vi "Fit Transform.vi"(7 "Type X":T1(ring), 8 "error in (no error)":errorcluster caption="entrée d'erreur (pas d'erreur)", 10 "y":string[][](array[string]), 11 "LabelBinarizer.lvclass":refnum<class "LabelBinarizer.lvclass">) -> (0 "error out":errorcluster caption="sortie d'erreur", 2 "Data":T2, 3 "LabelBinarizer.lvclass":refnum<class "LabelBinarizer.lvclass">)   [LabVIEW 2020, in "LabelBinarizer.lvclass"]
doc: "Fit label binarizer and transform multi-class labels to binary labels.\n\nThe output of transform is sometimes referred to as the 1-of-K coding scheme.\n\nReturns : \n\n- Y : array or CSR matrix of shape [n_samples, n_classes]\nShape will be [n_samples, 1] for binary problems."
uses:
  LabelBinarizer.lvclass
  LabelBinarizer.lvclass/LabelBinarizer.ctl
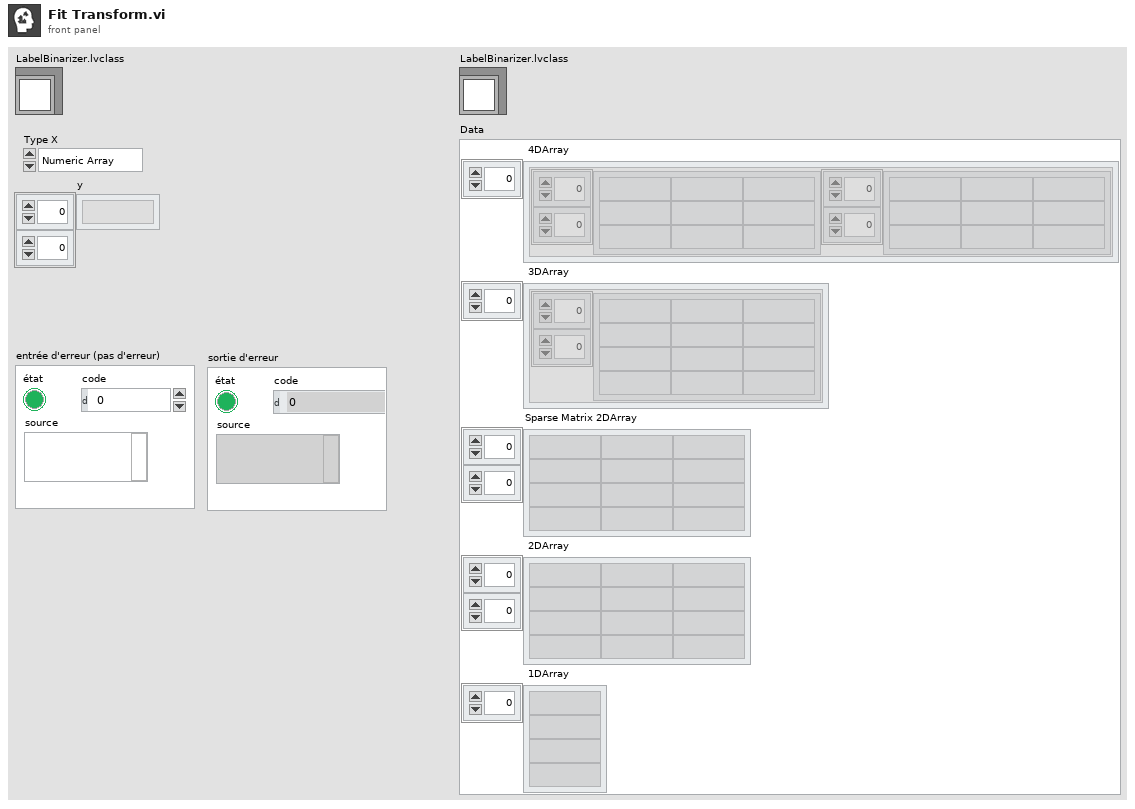
[diagram p1: front panel]
types:
  T1 = enum16{"Numeric Array", "String Array", "Sparse"}
  T2 = cluster{" 4DArray":cluster{"1":string[][], "2":string[][]}[], " 3DArray":cluster{"Tableau":string[][]}[], "Sparse Matrix 2DArray":string[][], " 2DArray":string[][], " 1DArray":string[]}
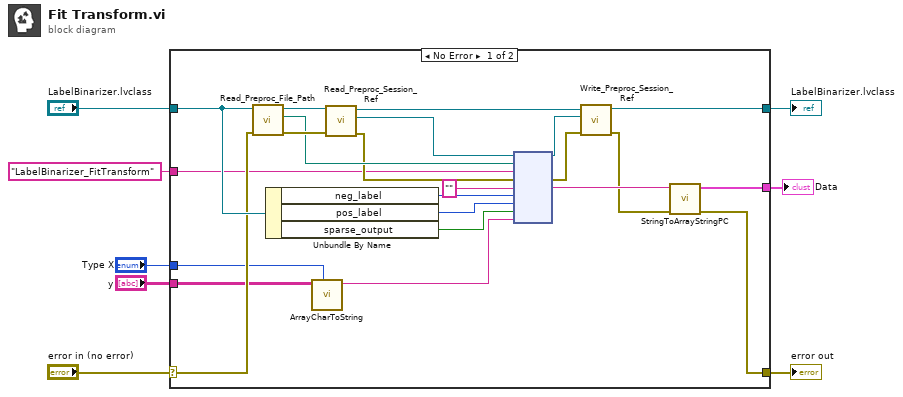
[diagram p0: block diagram]
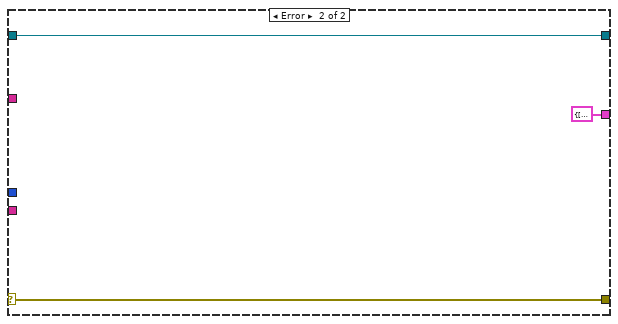
[diagram p2: hidden frame]
diagram:
  n1 = case shown="No Error" "error in (no error)" {
    selector: "error in (no error)" -> [w18 w34]
    tunnel: [w9 w34] -> w7
    tunnel: [w11 w33] -> w5
    tunnel: "LabelBinarizer.lvclass" -> [w19 w33]
    tunnel: "LabelBinarizer_FitTransform" ("Fonction") -> [w17 _]
    tunnel: [w10 T2 {" 4DArray"=[], " 3DArray"=[], "Sparse Matrix 2DArray"=[], " 2DArray"=[], " 1DArray"=[]} ("Data")] -> w3
    tunnel: "y" -> [w16 _]
    tunnel: "Type X" -> [w15 _]
    frame No Error {
      n2 = call-dynamic "Read_Preproc_File_Path.vi"("error in (no error)"=w18, "Python in"=w19) -> ("error out"=w30:errorcluster, "File_Path"=w27:path, "Python out"=w31:refnum<class "LabelBinarizer.lvclass">)  [unwired: 7 in]
      n3 = Unbundle By Name(w19) -> ("neg_label"=w22:i32, "pos_label"=w21:i32, "sparse_output"=w20:bool)
      n4 = call "ArrayCharToString.vi"("Type"=w15, "TAB"=w16) -> ("Instruction"=w14:string)  [unwired: 9 in]
      n5 = call-dynamic "Read_Preproc_Session_Ref.vi"("error in (no error)"=w30, "Python in"=w31) -> ("error out"=w26:errorcluster, "Session_ref"=w28:refnum<k35>, "Python out"=w29:refnum<class "LabelBinarizer.lvclass">)  [unwired: 7 in]
      n6 = node(w28, w27, w17, w26, "", w22, w21, w20, w14) -> (w24:refnum<k35>, w25:errorcluster, w13:string)  [unwired: 4 in, 2 out]
      n7 = call-dynamic "Write_Preproc_Session_Ref.vi"("error in (no error)"=w25, "Session_ref"=w24, "Python in"=w29) -> ("error out"=w12:errorcluster, "Python out"=w11:refnum<class "LabelBinarizer.lvclass">)  [unwired: 7 in]
      n8 = call "StringToArrayStringPC.vi"("sortie d'erreur"=w12, "Return value"=w13) -> ("sortie d'erreur"=w9:errorcluster, "Data"=w10:T2)  [unwired: 8 in]
    }
    frame Error {
    }
  }
  "error out" <- w7
  "LabelBinarizer.lvclass" <- w5
  "Data" <- w3
